vi "Create Double Commands.vi"(8 "Double Values":dbl[](array[numeric]), 11 "Commands":string) -> (3 "Result":string)   [LabVIEW 2014, in "Agilent MXA Series.lvlib"]
doc: "You can use this vi to create a command based on the input string and double values."
uses:
  Agilent MXA Series.lvlib
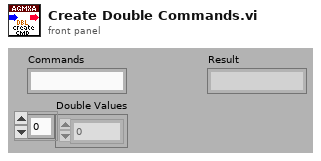
[diagram p1: front panel]
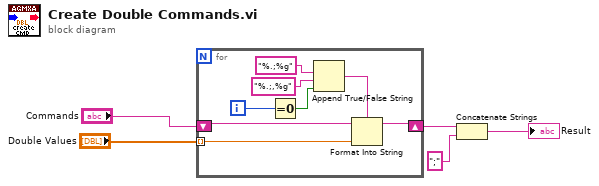
[diagram p0: block diagram]
diagram:
  n1 = for {
    tunnel: "Double Values" -> [w8] mode=indexing
    shift-right: [w6] -> w4
    shift-left: "Commands" -> [w7]
    i -> [w9]
    n2 = Equal To 0?(x=w9) -> (x = 0?=w10:bool)
    n3 = Append True/False String(1:w10, 2:"%.;,%g" ("format string"), 3:"%.;%g" ("format string")) -> (0:w13:string)  [unwired: 1 in]
    n4 = Format Into String(format string=w13, initial string=w7, w8) -> (resulting string=w6:string)  [unwired: 1 in, 1 out]
  }
  n5 = Concatenate Strings(w4, ";" ("string")) -> (→"Result":string)
